vi "CV_CB_main.vi"() -> ()   [LabVIEW 2021]
uses:
  C:/Users/User/Documents/Published_files/thorlabs_files/Thorlabs.MotionControl.Controls.dll
  thorlabs_files/Thorlabs.MotionControl.Controls.dll
  C:/Users/User/Documents/Published_files/thorlabs_files/ThorLabs.MotionControl.Benchtop.DCServoCLI.dll
  thorlabs_files/ThorLabs.MotionControl.Benchtop.DCServoCLI.dll
  C:/Users/User/Documents/Published_files/thorlabs_files/ThorLabs.MotionControl.KCube.DCServoCLI.dll
  thorlabs_files/ThorLabs.MotionControl.KCube.DCServoCLI.dll
  C:/Users/User/Documents/Published_files/thorlabs_files/Thorlabs.MotionControl.IntegratedStepperMotorsCLI.dll
  thorlabs_files/Thorlabs.MotionControl.IntegratedStepperMotorsCLI.dll
  <vilib>/Utility/file.llb/Read Delimited Spreadsheet (DBL).vi
  <vilib>/Utility/file.llb/Write Delimited Spreadsheet (DBL).vi
  <vilib>/ptbypt/NI_PtbyPt.lvlib
panel:
  in  "Use the last scan":bool
  out "Lumedica report 2":string
  in  "saveing method 2":string(combo)="SaveQueueImages"
  out "large_C":bool
  out "last Z":dbl format="%#.6g"
  in  "Pause Button":bool
  in  "Abort craniotomy":bool
  out "Going to perfrom a craniotomy":bool
  in  "Z-bias in pixels":dbl
  in  "feedrate (mm/s)":dbl=1.0
  out "TERMINATE":bool
  out "thickness":dbl
  out "calibration_pos":dbl[][](array[numeric])
  in  "Drilling type":i64(ring) items=["Constant remaining thickness", "Burr holes", "Constant trench depth"]
  in  "Refractive index":dbl=1.6
  in  "Previous Button":bool
  in  "Go to OCT site":bool
  in  "shut down":bool
  out "End":bool=TRUE
  out "Correction matrix":dbl[](array[numeric])
  out "Lumedica report":string
  in  "saveing method":string(combo)="SaveQueueImages"
  out "OCT_imaging_position":dbl[](array[numeric])
  in  "start OCT":bool
  out "OCT_on":bool
  out "X-stage Control":refnum<k24>
  out "X stage properties":refnum<k24>
  in  "LongTravelStageControl":refnum<k24>(container)
  out "Drill-Z-stage Control":refnum<k24>
  out "OCT-Z-stage-control":refnum<k24>
  out "Y-stage Control":refnum<k24>
  out "Y-stage properties":refnum<k24>
  out "Driller-Z-stage-Properties":refnum<k24>
  out "OCT-Z stage-properites":refnum<k24>
  in  "Trajectory":dbl[][](array[numeric])
  out "Velocity":T1(graph)
  out "position":T1(graph)
  in  "Driller Z- stage":refnum<k24>(container)
  in  "Y stage":refnum<k24>(container)
  in  "OCT Z-stage":refnum<k24>(container)
  # "Step Specified Controls"
  # "General Controls"
  # "Moving the stereotax to the OCT stage"
  # "OCT scanning"
  # "Moving to the surgery station"
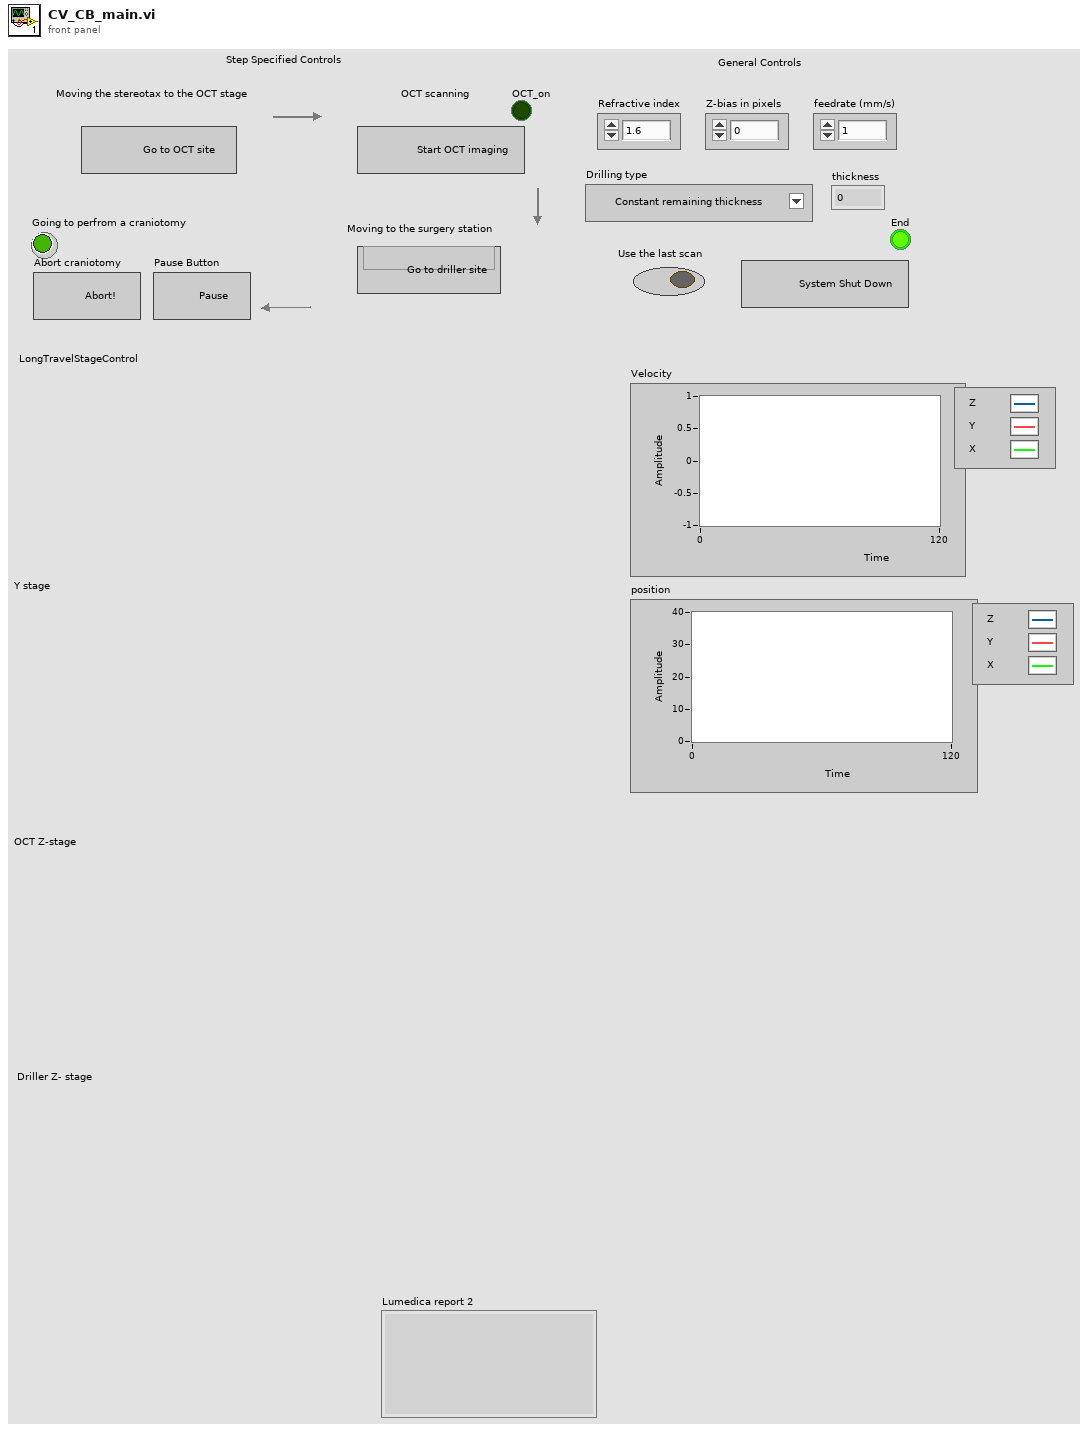
[diagram p1: front panel]
types:
  T1 = cluster{"[0]":dbl, "[1]":dbl, "[2]":dbl, "[3]":dbl, "[4]":dbl, "[5]":dbl, "[6]":dbl, "[7]":dbl, "[8]":dbl}
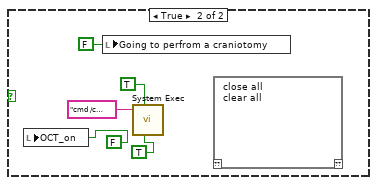
[diagram p2: hidden frame]
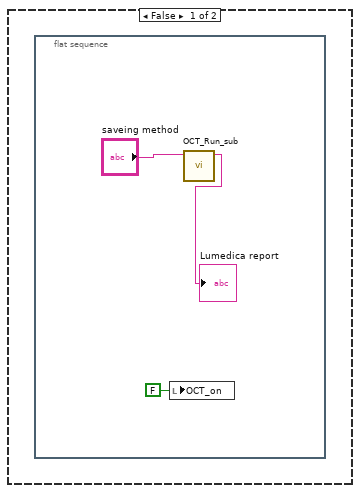
[diagram p5: hidden frame]
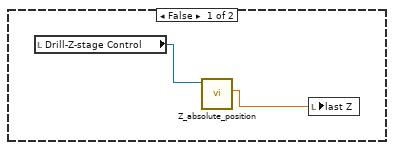
[diagram p9: hidden frame]
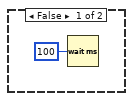
[diagram p10: hidden frame]
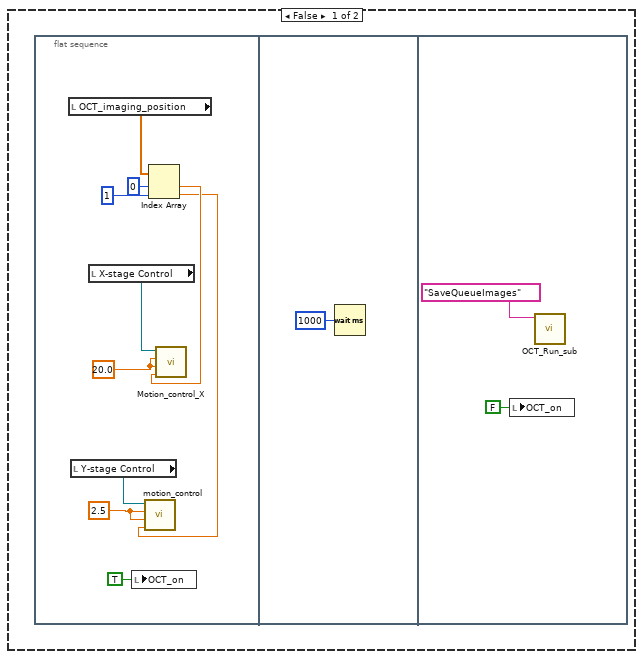
[diagram p12: hidden frame]
diagram:
  n1 = flat-sequence {
    frame #0 {
      # "Initiate all actuators"
      n2 = local write "End"(FALSE ("End")) -> ()
      n3 = property class="LongTravelStageControl"(reference="LongTravelStageControl", "SerialNumber"="45285094") -> (reference out=w25:refnum<k24>)  [unwired: 1 in, 1 out]
      n4 = property class="BenchtopDCServoControl"(reference="Y stage", "SerialNumber"="105278474") -> (reference out=w34:refnum<k24>)  [unwired: 1 in, 1 out]
      n5 = property class="KCubeDCServoControl"(reference="Driller Z- stage", "SerialNumber"="27260819") -> (reference out=w36:refnum<k24>)  [unwired: 1 in, 1 out]
      n6 = property class="KCubeDCServoControl"(reference="OCT Z-stage", "SerialNumber"="27261776") -> (reference out=w39:refnum<k24>)  [unwired: 1 in, 1 out]
      n7 = invoke class="LongTravelStageControl" method="CreateDevice"(reference=w25) -> (reference out=w24:refnum<k24>)  [unwired: 2 in, 2 out]
      n8 = invoke class="BenchtopDCServoControl" method="CreateDevice"(reference=w34) -> (reference out=w31:refnum<k24>)  [unwired: 2 in, 2 out]
      n9 = invoke class="KCubeDCServoControl" method="CreateDevice"(reference=w39) -> (reference out=w37:refnum<k24>)  [unwired: 2 in, 2 out]
      n10 = invoke class="KCubeDCServoControl" method="CreateDevice"(reference=w36) -> (reference out=w32:refnum<k24>)  [unwired: 2 in, 2 out]
      n11 = property class="LongTravelStageControl"(reference=w24) -> (reference out=w23:refnum<k24>, "Device"=w16:refnum<k24>)  [unwired: 1 in, 1 out]
      n12 = invoke class="IntegratedStepperMotor" method="SetBacklash"(reference=w16, "backlash"=0.002) -> ()  [unwired: 2 in, 4 out]
      n13 = property class="KCubeDCServoControl"(reference=w37) -> (reference out=w30:refnum<k24>, "Device"=w11:refnum<k24>)  [unwired: 1 in, 1 out]
      n14 = property class="BenchtopDCServoControl"(reference=w31) -> (reference out=w28:refnum<k24>, "BenchtopDCServo"=w14:refnum<k24>)  [unwired: 1 in, 1 out]
      n15 = invoke class="DCServoChannel" method="SetBacklash"(reference=w14, "backlash"=0.0) -> ()  [unwired: 2 in, 4 out]
      n16 = property class="KCubeDCServoControl"(reference=w32) -> (reference out=w29:refnum<k24>, "Device"=w27:refnum<k24>)  [unwired: 1 in, 1 out]
      n17 = invoke class="KCubeDCServo" method="SetBacklash"(reference=w27, "backlash"=0.007) -> ()  [unwired: 2 in, 4 out]
      n18 = invoke class="DCServoChannel" method="EnableDevice"(reference=w14) -> ()  [unwired: 2 in, 3 out]
      n19 = local write "OCT-Z stage-properites"(w30) -> ()
      n20 = local write "OCT-Z-stage-control"(w11) -> ()
      n21 = invoke class="KCubeDCServo" method="SetBacklash"(reference=w11, "backlash"=0.007) -> ()  [unwired: 2 in, 4 out]
      n22 = invoke class="IntegratedStepperMotor" method="EnableDevice"(reference=w16) -> ()  [unwired: 2 in, 3 out]
      n23 = local write "X stage properties"(w23) -> ()
      n24 = local write "X-stage Control"(w16) -> ()
      n25 = local write "Y-stage properties"(w28) -> ()
      n26 = local write "Y-stage Control"(w14) -> ()
      n27 = local write "Driller-Z-stage-Properties"(w29) -> ()
      n28 = local write "Drill-Z-stage Control"(w27) -> ()
    }
    frame #1 {
      # "Ready to take mouse to the imaging post"
      n29 = local read "Drill-Z-stage Control"() -> (w44:refnum<k24>)
      n30 = local write "OCT_on"(FALSE ("OCT_on")) -> ()
      n31 = call "motion control_Z.vi"("position"=0.0, "acceleration"=2.0, "maxVelocity"=2.0, ".NET Refnum in"=w44) -> ()  [unwired: 1 in, 1 out]
      n32 = call <vilib>:"System Exec.vi"("run minimized? (F)"=TRUE, "wait until completion? (T)"=TRUE, "command line"="cmd /c taskkill /IM OctEngine.exe") -> ()  [unwired: 5 in, 4 out]
      n33 = Two Button Dialog(message="Ready to move the mouse to OCT stage?", 1:"Nope! wait" ("F button name (\"Cancel\")"), 2:"Yes!" ("T button name (\"OK\")")) -> (T button?=w48:bool)
      n34 = while {
        tunnel: w48 -> [w52]
        stop <- w54 stop-if-true
        n35 = Or(x="Go to OCT site", y=w52) -> (x .or. y?=w54:bool)
      }
    }
    frame #2 {
      w68 = 3.0 ("maxVelocity")
      w73 = 20.0 ("maxVelocity")
      # "Move X actuator to 285mm"
      n36 = local read "X-stage Control"() -> (w74:refnum<k24>)
      n37 = call <vilib>:"Application Directory.vi"() -> ("Application Directory"=w62:path)
      n38 = local read "Y-stage Control"() -> (w70:refnum<k24>)
      n39 = local read "OCT-Z-stage-control"() -> (w69:refnum<k24>)
      n40 = Build Path(base path=w62, name or relative path=path "temp_files/Calibration_imaging_position.txt" ("file path (dialog if empty)")) -> (appended path=w63:path)
      n41 = call-poly <vilib>:"Read Delimited Spreadsheet.vi"("file path (dialog if empty)"=w63) -> ("all rows"=w60:dbl[][])  [unwired: 9 in, 5 out]
      n42 = local write "calibration_pos"(w60) -> ()
      n43 = Index Array(array=w60, index (row)=0, index (col)=1 ("disabled index (col)")) -> (element=w55:dbl)
      n44 = Index Array(array=w60, index (row)=0, index (col)=0 ("disabled index (col)")) -> (element=w61:dbl)
      n45 = call "Motion_control_X.vi"(".NET Refnum in"=w74, "maxVelocity"=w73, "acceleration"=w73, "position"=w61) -> ()  [unwired: 6 in, 1 out]
      n46 = Index Array(array=w60, index (row)=0 ("disabled index (row)"), index (col)=2 ("disabled index (col)")) -> (element=w66:dbl)
      n47 = call "motion_control.vi"("position"=w55, "acceleration"=5.0, "maxVelocity"=2.5, ".NET Refnum in"=w70) -> ()  [unwired: 1 in, 1 out]
      n48 = call "motion control_Z.vi"("position"=w66, "acceleration"=w68, "maxVelocity"=w68, ".NET Refnum in"=w69) -> ()  [unwired: 1 in, 1 out]
    }
    frame #3 {
      n49 = Two Button Dialog(message="What is the size of your FOV?", 1:"Less than 5 mm2" ("F button name (\"Cancel\")"), 2:"More than 5 mm2" ("T button name (\"OK\")")) -> (T button?=w75:bool)
      n50 = local write "large_C"(w75) -> ()
    }
    frame #4 {
      # "Manually adjust the imaging setp"
      n51 = while {
        stop <- w82 stop-if-true
        n52 = One Button Dialog(message="Adjust the sample position under the scanner and hit \"Take OCT image\" in labview", button name ("OK")="OK") -> (true=w82:bool)
      }
      n53 = Wait (ms)(milliseconds to wait=u32 1000) -> ()  [unwired: 1 out]
    }
    frame #5 {
      # "Show the USB camera and the FOV"
      n54 = local read "large_C"() -> (w84:bool)
      n55 = call <vilib>:"Application Directory.vi"() -> ("Application Directory"=w85:path)
      n56 = Boolean To (0,1)(Boolean=w84) -> (0, 1=w83:i16)
      n57 = script code="load([path,'\\temp_files\\pilot.mat'])\nif large>0\n     Xoff=110; Yoff=80;\nelse\n     Xoff=0; Yoff=0;\nend\nvid = videoinput('winvideo',OCT_cam);\nvidRes = vid.VideoResolution;\nnBands = vid.NumberOfBands; \n\nhFig=figure('Renderer', 'painters', 'Position', [1100 200 vidRes(1)/2+2*Xoff vidRes(2)]);\nhAxes = axes(hFig);\nhImage = image(hAxes, zeros(vidRes(2), vidRes(1)/2+2*Xoff, nBands)); \n\nsetappdata(hImage,'UpdatePreviewWindowFcn',@mypreview_fnc);\n\npreview(vid, hImage); \n% adding the OCT image boarders to the video\nhold on\ntext(-40,-35,'Make sure your ROI is in the green rectangle. if it is, just close the window','FontWeight','bold','FontSize',12)\n\nline([pilot(4,1)-Xoff pilot(1,1)+Xoff], [pilot(4,2)-Yoff pilot(1,2)-Yoff],'Color','g','LineWidth',3);\nline([pilot(3,1)-Xoff pilot(4,1)-Xoff], [pilot(3,2)+Yoff pilot(4,2)-Yoff],'Color','g','LineWidth',3);\nline([pilot(2,1)+Xoff pilot(3,1)-Xoff], [pilot(2,2)+Yoff pilot(3,2)+Yoff],'Color','g','LineWidth',3);\nline([pilot(1,1)+Xoff pilot(2,1)+Xoff], [pilot(1,2)-Yoff pilot(2,2)+Yoff],'Color','g','LineWidth',3);\n\n\nclear camObject;"("path"=w85, "large"=w83) -> ()  [unwired: 1 in, 1 out]
    }
    frame #6 {
      # "Acquire the stage positions during imaging"
      n58 = case shown="False" "Use the last scan" {
        frame False {
          n59 = while {
            tunnel: [w100] -> w88
            tunnel: [w99] -> w87
            tunnel: [w98] -> w94
            stop <- w96 stop-if-true
            n60 = local read "OCT-Z-stage-control"() -> (w101:refnum<k24>)
            n61 = local read "Y-stage Control"() -> (w102:refnum<k24>)
            n62 = local read "X-stage Control"() -> (w103:refnum<k24>)
            n63 = local read "TERMINATE"() -> (w95:bool)
            n64 = call "Y_absolute_position.vi"(".NET Refnum in"=w102) -> ("Numeric"=w99:dbl)  [unwired: 9 in, 1 out]
            n65 = Or(x=w95, y="start OCT") -> (x .or. y?=w96:bool)
            n66 = call "X-absolute_position.vi"(".NET Refnum in"=w103) -> ("Numeric"=w100:dbl)  [unwired: 9 in, 1 out]
            n67 = call "Z_absolute_position.vi"(".NET Refnum in"=w101) -> ("Numeric"=w98:dbl)  [unwired: 9 in, 1 out]
          }
          n68 = local write "OCT_on"(TRUE ("OCT_on")) -> ()
          n69 = Build Array(w88, w87, w94) -> (w93:dbl[])
          n70 = local write "OCT_imaging_position"(w93) -> ()
          n71 = call <vilib>:"Application Directory.vi"() -> ("Application Directory"=w91:path)
          n72 = Build Path(base path=w91, name or relative path=path "temp_files/imaging_position.txt" ("file path (dialog if empty)")) -> (appended path=w89:path)
          n73 = call-poly <vilib>:"Write Delimited Spreadsheet.vi"("file path (dialog if empty)"=w89, "1D data"=w93) -> ()  [unwired: 12 in, 2 out]
        }
        frame True {
        }
      }
    }
    frame #7 {
      n74 = local read "Use the last scan"() -> (w104:bool)
      n75 = case shown="False" w104 {
        frame False {
          # "Take the OCT image"
          n76 = local read "large_C"() -> (w105:bool)
          n77 = case shown="True" w105 {
            frame False {
              n78 = flat-sequence {
                frame #0 {
                  n79 = local write "OCT_on"(FALSE ("OCT_on")) -> ()
                  n80 = call "OCT_Run_sub.vi"("saveing method"="saveing method") -> ("Lumedica report"=→"Lumedica report":string)  [unwired: 10 in]
                }
              }
            }
            frame True {
              w110 = -2.25 ("element")
              w111 = 2.25 ("element")
              w113 = -2.0 ("element")
              w114 = 2.0 ("element")
              # "Shifts need in Y direction for each\nquarter of the big scan with respect to the center"
              # "Shifts need in X direction for each\nquarter of the big scan with respect to the center"
              # "make sure it is 4"
              n81 = Build Array(w111, w110, w110, w111) -> (w109:dbl[])
              n82 = Build Array(w114, w114, w113, w113) -> (w112:dbl[])
              n83 = for {
                N: 4 -> [_]
                tunnel: w112 -> [w118] mode=indexing
                tunnel: w109 -> [w117] mode=indexing
                n84 = flat-sequence {
                  tunnel: w118 -> [w123]
                  tunnel: w117 -> [w120]
                  frame #0 {
                    w128 = 2.0 ("maxVelocity")
                    w129 = 2.0 ("maxVelocity")
                    # "move to the target quarter"
                    n85 = local read "OCT_imaging_position"() -> (w127:dbl[])
                    n86 = local read "X-stage Control"() -> (w131:refnum<k24>)
                    n87 = local read "Y-stage Control"() -> (w130:refnum<k24>)
                    n88 = Index Array(array=w127, index #1=0 ("index"), index #2=1 ("index")) -> (element #1=w124:dbl, element #2=w121:dbl)
                    n89 = Add(x=w124, y=w123) -> (x+y=w122:dbl)
                    n90 = Add(x=w121, y=w120) -> (x+y=w119:dbl)
                    n91 = call "motion_control.vi"("position"=w119, "acceleration"=w128, "maxVelocity"=w128, ".NET Refnum in"=w130) -> ()  [unwired: 1 in, 1 out]
                    n92 = call "Motion_control_X.vi"(".NET Refnum in"=w131, "maxVelocity"=w129, "acceleration"=w129, "position"=w122) -> ()  [unwired: 6 in, 1 out]
                  }
                  frame #1 {
                    n93 = Wait (ms)(milliseconds to wait=u32 1000) -> ()  [unwired: 1 out]
                  }
                  frame #2 {
                    # "Take OCT stack of the quarter"
                    n94 = call "OCT_Run_sub.vi"("saveing method"="saveing method 2") -> ("Lumedica report"=→"Lumedica report 2":string)  [unwired: 10 in]
                  }
                }
              }
              n95 = local write "OCT_on"(FALSE ("OCT_on")) -> ()
            }
          }
        }
        frame True {
        }
      }
    }
    frame #8 {
      # "Try to close the opened video windoe"
      # "Close lumedica and open video windows"
      n96 = script code="close all"() -> ()  [unwired: 1 in, 1 out]
      n97 = call <vilib>:"System Exec.vi"("run minimized? (F)"=TRUE, "wait until completion? (T)"=TRUE, "command line"="cmd /c taskkill /IM OctEngine.exe") -> ()  [unwired: 5 in, 4 out]
    }
    frame #9 {
      # "This address should be tha same as where OCT saves scans"
      # "Calculating the first path"
      n98 = local read "Z-bias in pixels"() -> (w141:dbl)
      n99 = local read "large_C"() -> (w139:bool)
      n100 = call "File Dialog2"() -> ("selected path"=w140:path)  [unwired: 12 in, 3 out]
      n101 = local write "Going to perfrom a craniotomy"(TRUE ("Going to perfrom a craniotomy")) -> ()
      n102 = local read "Drilling type"() -> (w145:i64)
      n103 = local read "calibration_pos"() -> (w142:dbl[][])
      n104 = call "Calculate_drilling_path.vi"("calibration_pos"=w142, "Refractive index of the sample"="Refractive index", "Drilling type"=w145, "Large_C"=w139, "Z-bias in pixels"=w141, "Drilling path"=w140, "file path (dialog if empty)"=path "C:/Users/Public/Documents/Lumedica/OctEngine/Data") -> ("depth"=→"thickness":dbl)  [unwired: 4 in]
    }
    frame #10 {
      n105 = disable-structure shown="Disabled" {
        frame Disabled {
          n106 = Path To String(path=path "C:/Users/Public/Documents/Lumedica/OctEngine/Data" ("file path (dialog if empty)")) -> (string=w155:string)
          n107 = Concatenate Strings("cmd /k explorer.exe  " ("string"), w155, "\\figures" ("string")) -> (w153:string)
          n108 = call <vilib>:"System Exec.vi"("run minimized? (F)"=TRUE, "wait until completion? (T)"=FALSE, "command line"=w153) -> ()  [unwired: 5 in, 4 out]
        }
        frame Enabled {
        }
      }
      n109 = Two Button Dialog(message="Ready to move the mouse to drilling  stage?", 1:"Nope! wait" ("F button name (\"Cancel\")"), 2:"Yes!" ("T button name (\"OK\")")) -> (T button?=w147:bool)
      n110 = while {
        tunnel: w147 -> [w159]
        stop <- w160 stop-if-true
        n111 = Or(x=w159, y="Previous Button") -> (x .or. y?=w160:bool)
      }
    }
    frame #11 {
      w166 = 20.0 ("maxVelocity")
      # "Move the stage to the drilling site"
      n112 = local read "Y-stage Control"() -> (w162:refnum<k24>)
      n113 = local read "X-stage Control"() -> (w161:refnum<k24>)
      n114 = call "Motion_control_X.vi"(".NET Refnum in"=w161, "maxVelocity"=w166, "acceleration"=w166, "position"=17.0) -> ()  [unwired: 6 in, 1 out]
      n115 = call "motion_control.vi"("position"=10.0, "acceleration"=5.0, "maxVelocity"=2.5, ".NET Refnum in"=w162) -> ()  [unwired: 1 in, 1 out]
    }
    frame #12 {
      # "turn on the drill camera"
      n116 = call <vilib>:"Application Directory.vi"() -> ("Application Directory"=w168:path)
      n117 = script code="load([path,'\\temp_files\\pilot.mat'])\ncrop_pixels=100;\nvid = videoinput('winvideo',Drill_cam);\nvidInfo = imaqhwinfo(vid);\nvidRes = vid.VideoResolution;\nnBands = vid.NumberOfBands; \nhFig=figure('Renderer', 'painters', 'Position', [1200 200 vidRes(1)/2 vidRes(2)/2]);\nhAxes = axes(hFig);\nhImage = image(hAxes, zeros(vidRes(2), vidRes(1), nBands)); \n%setappdata(hImage,'UpdatePreviewWindowFcn',@mypreview_fnc);\npreview(vid, hImage); \n% adding the OCT image boarders to the video\nhold on\ntext(-40,-35,'Drilling FOV','FontWeight','bold','FontSize',12)\n\nclear camObject;"("path"=w168) -> ()  [unwired: 1 in, 1 out]
    }
    frame #13 {
      # "Ready for drilling!"
      n118 = while {
        stop <- w171 stop-if-true
        n119 = One Button Dialog(message="Drop sailine on top of  the skull , TURN ON THE DRILLERTand press ok when you are ready", button name ("OK")="OK") -> (true=w171:bool)
      }
    }
    frame #14 {
      n120 = while {
        stop <- w180 stop-if-true
        n121 = flat-sequence {
          tunnel: [w181] -> w179
          tunnel: w179 -> [w185]
          tunnel: [w186] -> w178
          tunnel: [w185] -> w176
          tunnel: w178 -> [w204]
          tunnel: [w203] -> w177
          tunnel: w176 -> [w203]
          tunnel: w177 -> [w209]
          tunnel: [w208] -> w175
          tunnel: [w207] -> w174
          tunnel: w175 -> [w224]
          tunnel: w174 -> [w223]
          tunnel: [w258] -> w173
          tunnel: w173 -> [w262]
          tunnel: [w262] -> w172
          frame #0 {
            # "read the calculated drilling path"
            n122 = call <vilib>:"Application Directory.vi"() -> ("Application Directory"=w184:path)
            n123 = Build Path(base path=w184, name or relative path=path "temp_files/C_TD_path.txt" ("file path (dialog if empty)")) -> (appended path=w183:path)
            n124 = call-poly <vilib>:"Read Delimited Spreadsheet.vi"("file path (dialog if empty)"=w183) -> ("all rows"=w181:dbl[][])  [unwired: 9 in, 5 out]
          }
          frame #1 {
            w197 = 2.0 ("maxVelocity")
            w201 = 20.0 ("maxVelocity")
            # "Move to the first poin-0.5 mm up"
            n125 = local read "Drill-Z-stage Control"() -> (w199:refnum<k24>)
            n126 = Index Array(array=w185, index (row)=0) -> (element=w193:dbl[])  [unwired: 1 in]
            n127 = local read "X-stage Control"() -> (w202:refnum<k24>)
            n128 = Index Array(array=w193, index #1=0 ("index"), index #2=1 ("index"), index #3=2 ("index")) -> (element #1=w187:dbl, element #2=w188:dbl, element #3=w186:dbl)
            n129 = Subtract(x=w186, y=0.5) -> (x-y=w200:dbl)
            n130 = local read "Y-stage Control"() -> (w196:refnum<k24>)
            n131 = call "motion control_Z.vi"("position"=w200, "acceleration"=w197, "maxVelocity"=w197, ".NET Refnum in"=w199) -> ()  [unwired: 1 in, 1 out]
            n132 = call "motion_control.vi"("position"=w188, "acceleration"=5.0, "maxVelocity"=2.5, ".NET Refnum in"=w196) -> ()  [unwired: 1 in, 1 out]
            n133 = call "Motion_control_X.vi"(".NET Refnum in"=w202, "maxVelocity"=w201, "acceleration"=w201, "position"=w187) -> ()  [unwired: 6 in, 1 out]
          }
          frame #2 {
            w205 = 0.25 ("maxVelocity")
            # "Drill down the first point"
            n134 = local read "Drill-Z-stage Control"() -> (w206:refnum<k24>)
            n135 = call "motion control_Z.vi"("position"=w204, "acceleration"=w205, "maxVelocity"=w205, ".NET Refnum in"=w206) -> ()  [unwired: 1 in, 1 out]
          }
          frame #3 {
            # "calculate speeds and positions"
            n136 = disable-structure shown="Disabled" {
              disable-tunnel: w209 -> [w211 _]
              frame Disabled {
                n137 = script code="ratio=1;\ndata=C_TD_path(:,1:3)';\n[q, qd, qdd, tvec, pp] = trapveltraj(data,length(C_TD_path));\ncoef=pp{1,1}.coefs;\naccX=2*coef(4:9:end,1);\naccY=2*coef(5:9:end,1);\naccZ=2*coef(6:9:end,1);\nmVelX=coef(7:9:end,2);\nmVelY=coef(8:9:end,2);\nmVelZ=coef(9:9:end,2);\nmVel=ratio*abs([mVelX mVelY mVelZ]);\nmVel(mVel<0.02)=0.02;\nacc=(ratio^2)*abs([accX accY accZ]);\nacc(acc<0.02)=0.02;\nTime=pp{1,1}.breaks;\nTime=Time(2:3:end);\nWTime=Time(2:end)-Time(1:end-1);\nsteps=length(WTime);\ndata=data(:,2:end)';"("C_TD_path"=w211) -> ("mVel"=w212:dbl[][], "acc"=w213:dbl[][], "data"=w210:dbl[][])  [unwired: 1 in, 2 out]
                n138 = call <vilib>:"Application Directory.vi"() -> ("Application Directory"=w222:path)
                n139 = call <vilib>:"Application Directory.vi"() -> ("Application Directory"=w221:path)
                n140 = call <vilib>:"Application Directory.vi"() -> ("Application Directory"=w220:path)
                n141 = Build Path(base path=w222, name or relative path=path "temp_files/F_a_log.txt" ("file path (dialog if empty)")) -> (appended path=w214:path)
                n142 = Build Path(base path=w221, name or relative path=path "temp_files/F_p_log.txt" ("file path (dialog if empty)")) -> (appended path=w216:path)
                n143 = Build Path(base path=w220, name or relative path=path "temp_files/F_v_log.txt" ("file path (dialog if empty)")) -> (appended path=w219:path)
                n144 = call-poly <vilib>:"Write Delimited Spreadsheet.vi"("file path (dialog if empty)"=w219, "2D data"=w212) -> ()  [unwired: 12 in, 2 out]
                n145 = call-poly <vilib>:"Write Delimited Spreadsheet.vi"("file path (dialog if empty)"=w214, "2D data"=w213) -> ()  [unwired: 12 in, 2 out]
                n146 = call-poly <vilib>:"Write Delimited Spreadsheet.vi"("file path (dialog if empty)"=w216, "2D data"=w210) -> ()  [unwired: 12 in, 2 out]
              }
              frame Enabled {
              }
            }
            n147 = script code="data=C_TD_path(:,1:3)';\ndata=data(:,2:end)';\nsteps=length(data);"("C_TD_path"=w209) -> ("steps"=w208:dbl, "data"=w207:dbl[][])  [unwired: 1 in, 1 out]
          }
          frame #4 {
            # "actuators moving"
            n148 = for {
              N: w224 -> [_]
              tunnel: w223 -> [w234] mode=indexing
              stop <- "Abort craniotomy" stop-if-true
              n149 = case shown="True" "Pause Button" {
                frame False {
                  n150 = local read "Drill-Z-stage Control"() -> (w239:refnum<k24>)
                  n151 = call "Z_absolute_position.vi"(".NET Refnum in"=w239) -> ("Numeric"=w238:dbl)  [unwired: 9 in, 1 out]
                  n152 = local write "last Z"(w238) -> ()
                }
                frame True {
                  w240 = 2.0 ("maxVelocity")
                  # "bring driller up for the moment"
                  n153 = flat-sequence {
                    frame #0 {
                      n154 = while {
                        stop <- w247 stop-if-true
                        n155 = One Button Dialog(message="Are you ready to go back?", button name ("OK")="Yup!") -> (true=w247:bool)
                      }
                    }
                    frame #1 {
                      w251 = 1.1 ("maxVelocity")
                      n156 = local read "Drill-Z-stage Control"() -> (w249:refnum<k24>)
                      n157 = local read "last Z"() -> (w250:dbl)
                      n158 = call "motion control_Z.vi"("position"=w250, "acceleration"=w251, "maxVelocity"=w251, ".NET Refnum in"=w249) -> ()  [unwired: 1 in, 1 out]
                    }
                  }
                  n159 = local read "Drill-Z-stage Control"() -> (w245:refnum<k24>)
                  n160 = call "Z_absolute_position.vi"(".NET Refnum in"=w245) -> ("Numeric"=w243:dbl, ".NET Refnum out"=w244:refnum<k24>)  [unwired: 9 in]
                  n161 = Subtract(x=w243, y=10.0) -> (x-y=w241:dbl)
                  n162 = call "motion control_Z.vi"("position"=w241, "acceleration"=w240, "maxVelocity"=w240, ".NET Refnum in"=w244) -> ()  [unwired: 1 in, 1 out]
                }
              }
              n163 = local read "Drill-Z-stage Control"() -> (w230:refnum<k24>)
              n164 = local read "feedrate (mm/s)"() -> (w227:dbl)
              n165 = local read "X-stage Control"() -> (w229:refnum<k24>)
              n166 = local read "Y-stage Control"() -> (w228:refnum<k24>)
              n167 = Index Array(array=w234, index #1=0 ("index"), index #2=1 ("index"), index #3=2 ("index")) -> (element #1=w233:dbl, element #2=w232:dbl, element #3=w231:dbl)
              n168 = call "motion_control.vi"("position"=w232, "acceleration"=w227, "maxVelocity"=w227, ".NET Refnum in"=w228) -> ()  [unwired: 1 in, 1 out]
              n169 = call "Motion_control_X.vi"(".NET Refnum in"=w229, "maxVelocity"=w227, "acceleration"=w227, "position"=w233) -> ()  [unwired: 6 in, 1 out]
              n170 = call "motion control_Z.vi"("position"=w231, "acceleration"=w227, "maxVelocity"=w227, ".NET Refnum in"=w230) -> ()  [unwired: 1 in, 1 out]
            }
          }
          frame #5 {
            w254 = 2.0 ("acceleration")
            # "Move up the drillbit after finishing"
            n171 = local read "Drill-Z-stage Control"() -> (w257:refnum<k24>)
            n172 = call "Z_absolute_position.vi"(".NET Refnum in"=w257) -> ("Numeric"=w253:dbl, ".NET Refnum out"=w256:refnum<k24>)  [unwired: 9 in]
            n173 = Subtract(x=w253, y=10.0) -> (x-y=w255:dbl)
            n174 = call "motion control_Z.vi"("position"=w255, "acceleration"=w254, "maxVelocity"=w254, ".NET Refnum in"=w256) -> ()  [unwired: 1 in, 1 out]
          }
          frame #6 {
            # "Asking if extra craniotomies are needed"
            n175 = Two Button Dialog(message="would you like to perform another craniotomy?", 1:"Nope. Done!" ("F button name (\"Cancel\")"), 2:"Yes!" ("T button name (\"OK\")")) -> (T button?=w258:bool)
            n176 = local write "Going to perfrom a craniotomy"(w258) -> ()
          }
          frame #7 {
            n177 = case shown="True" w262 {
              frame False {
                n178 = Wait (ms)(milliseconds to wait=u32 100) -> ()  [unwired: 1 out]
              }
              frame True {
                n179 = flat-sequence {
                  tunnel: [w266] -> w264
                  tunnel: w264 -> [w268]
                  frame #0 {
                    n180 = call "File Dialog"("prompt"="Choose the drilling path") -> ("selected path"=w266:path)  [unwired: 11 in, 3 out]
                  }
                  frame #1 {
                    n181 = local read "Z-bias in pixels"() -> (w272:dbl)
                    n182 = local read "large_C"() -> (w267:bool)
                    n183 = local read "Drilling type"() -> (w270:i64)
                    n184 = local read "Refractive index"() -> (w273:dbl)
                    n185 = local read "calibration_pos"() -> (w274:dbl[][])
                    n186 = call "Calculate_drilling_path.vi"("calibration_pos"=w274, "Refractive index of the sample"=w273, "Drilling type"=w270, "Large_C"=w267, "Z-bias in pixels"=w272, "Drilling path"=w268, "file path (dialog if empty)"=path "C:/Users/Public/Documents/Lumedica/OctEngine/Data") -> ("depth"=w271:dbl)  [unwired: 4 in]
                    n187 = local write "thickness"(w271) -> ()
                  }
                }
              }
            }
          }
        }
        n188 = Not(x=w172) -> (.not. x?=w180:bool)
      }
    }
    frame #15 {
      w275 = 2.0 ("position")
      n189 = local read "Drill-Z-stage Control"() -> (w277:refnum<k24>)
      n190 = call "motion control_Z.vi"("position"=0.0 ("maxVelocity"), "acceleration"=w275, "maxVelocity"=w275, ".NET Refnum in"=w277) -> ()  [unwired: 1 in, 1 out]
    }
    frame #16 {
      n191 = Two Button Dialog(message="Would you like to check the drilled path", 1:"No" ("F button name (\"Cancel\")"), 2:"Yes!" ("T button name (\"OK\")")) -> (T button?=w278:bool)
      n192 = case shown="True" w278 {
        frame False {
        }
        frame True {
          n193 = local read "large_C"() -> (w282:bool)
          n194 = case shown="True" w282 {
            frame False {
              n195 = flat-sequence {
                frame #0 {
                  w291 = 2.5 ("maxVelocity")
                  w292 = 20.0 ("maxVelocity")
                  n196 = local read "OCT_imaging_position"() -> (w288:dbl[])
                  n197 = local read "Y-stage Control"() -> (w289:refnum<k24>)
                  n198 = local read "X-stage Control"() -> (w290:refnum<k24>)
                  n199 = local write "OCT_on"(TRUE ("OCT_on")) -> ()
                  n200 = Index Array(array=w288, index #1=0 ("index"), index #2=1 ("index")) -> (element #1=w285:dbl, element #2=w284:dbl)
                  n201 = call "motion_control.vi"("position"=w284, "acceleration"=w291, "maxVelocity"=w291, ".NET Refnum in"=w289) -> ()  [unwired: 1 in, 1 out]
                  n202 = call "Motion_control_X.vi"(".NET Refnum in"=w290, "maxVelocity"=w292, "acceleration"=w292, "position"=w285) -> ()  [unwired: 6 in, 1 out]
                }
                frame #1 {
                  n203 = Wait (ms)(milliseconds to wait=u32 1000) -> ()  [unwired: 1 out]
                }
                frame #2 {
                  n204 = local write "OCT_on"(FALSE ("OCT_on")) -> ()
                  n205 = call "OCT_Run_sub.vi"("saveing method"="SaveQueueImages") -> ()  [unwired: 10 in, 1 out]
                }
              }
            }
            frame True {
              w299 = -2.25 ("element")
              w300 = 2.25 ("element")
              w301 = -2.0 ("element")
              w302 = 2.0 ("element")
              n206 = Build Array(w300, w299, w299, w300) -> (w297:dbl[])
              n207 = Build Array(w302, w302, w301, w301) -> (w298:dbl[])
              n208 = for {
                N: 4 -> [_]
                tunnel: w298 -> [w305] mode=indexing
                tunnel: w297 -> [w304] mode=indexing
                n209 = flat-sequence {
                  tunnel: w305 -> [w310]
                  tunnel: w304 -> [w308]
                  frame #0 {
                    w317 = 20.0 ("acceleration")
                    w318 = 2.5 ("acceleration")
                    n210 = local read "OCT_imaging_position"() -> (w314:dbl[])
                    n211 = local read "Y-stage Control"() -> (w316:refnum<k24>)
                    n212 = local read "X-stage Control"() -> (w315:refnum<k24>)
                    n213 = Index Array(array=w314, index #1=0 ("index"), index #2=1 ("index")) -> (element #1=w311:dbl, element #2=w307:dbl)
                    n214 = Add(x=w307, y=w308) -> (x+y=w306:dbl)
                    n215 = Add(x=w311, y=w310) -> (x+y=w309:dbl)
                    n216 = call "motion_control.vi"("position"=w306, "acceleration"=w318, "maxVelocity"=w318, ".NET Refnum in"=w316) -> ()  [unwired: 1 in, 1 out]
                    n217 = call "Motion_control_X.vi"(".NET Refnum in"=w315, "maxVelocity"=w317, "acceleration"=w317, "position"=w309) -> ()  [unwired: 6 in, 1 out]
                  }
                  frame #1 {
                    n218 = Wait (ms)(milliseconds to wait=u32 1000) -> ()  [unwired: 1 out]
                  }
                  frame #2 {
                    n219 = call "OCT_Run_sub.vi"() -> ()  [unwired: 11 in, 1 out]
                  }
                }
              }
              n220 = local write "OCT_on"(TRUE ("OCT_on")) -> ()
            }
          }
        }
      }
    }
    frame #17 {
      n221 = script code="clear camObject;\nclose all\nclearvars\npack;\nclear all"() -> ()  [unwired: 1 in, 1 out]
    }
    frame #18 {
      n222 = local write "OCT_on"(FALSE ("OCT_on")) -> ()
      n223 = local write "End"(TRUE) -> ()
    }
  }
  n224 = local read "OCT-Z stage-properites"() -> (w2:refnum<k24>)
  n225 = local read "OCT-Z stage-properites"() -> (w4:refnum<k24>)
  n226 = local read "X stage properties"() -> (w1:refnum<k24>)
  n227 = local read "Y-stage properties"() -> (w3:refnum<k24>)
  n228 = flat-sequence {
    tunnel: w4 -> [w328]
    tunnel: w3 -> [w327]
    tunnel: [w326] -> w10
    tunnel: [w330] -> w9
    tunnel: [w329] -> w8
    tunnel: w2 -> [w326]
    tunnel: [w325] -> w7
    tunnel: [w324] -> w6
    tunnel: w1 -> [w323]
    tunnel: [w322] -> w5
    tunnel: w10 -> [w368]
    tunnel: w9 -> [w369]
    tunnel: w8 -> [w370]
    tunnel: w7 -> [w367]
    tunnel: w6 -> [w366]
    tunnel: w5 -> [w365]
    frame #0 {
      n229 = while {
        tunnel: [w352] -> w330
        tunnel: w328 -> [w352]
        tunnel: w327 -> [w351]
        tunnel: [w351] -> w329
        tunnel: [w341] -> w325 mode=indexing
        tunnel: [w340] -> w324 mode=indexing
        tunnel: w323 -> [w339]
        tunnel: [w339] -> w322
        stop <- w331 stop-if-true
        w337 = u32 250 ("milliseconds to wait")
        w346 = 0.0 ("initial condition")
        n230 = local read "Drill-Z-stage Control"() -> (w342:refnum<k24>)
        n231 = local read "X-stage Control"() -> (w338:refnum<k24>)
        n232 = local read "Y-stage Control"() -> (w343:refnum<k24>)
        n233 = local read "End"() -> (w333:bool)
        n234 = call "Y_absolute_position.vi"(".NET Refnum in"=w343) -> ("Numeric"=w345:dbl)  [unwired: 9 in, 1 out]
        n235 = call "Z_absolute_position.vi"(".NET Refnum in"=w342) -> ("Numeric"=w344:dbl)  [unwired: 9 in, 1 out]
        n236 = call "X-absolute_position.vi"(".NET Refnum in"=w338) -> ("Numeric"=w335:dbl)  [unwired: 9 in, 1 out]
        n237 = Or(x="shut down", y=w333) -> (x .or. y?=w331:bool)
        "TERMINATE" <- w331
        n238 = case shown="False" w331 {
          frame False {
          }
          frame True {
            n239 = local write "OCT_on"(FALSE ("OCT_on")) -> ()
            n240 = local write "Going to perfrom a craniotomy"(FALSE ("Going to perfrom a craniotomy")) -> ()
            n241 = call <vilib>:"System Exec.vi"("run minimized? (F)"=TRUE, "wait until completion? (T)"=TRUE, "command line"="cmd /c taskkill /IM OctEngine.exe") -> ()  [unwired: 5 in, 4 out]
            n242 = script code="close all\nclear all"() -> ()  [unwired: 1 in, 1 out]
          }
        }
        n243 = call <vilib>:"Derivative x(t) PtByPt.vi"("dt"=w337, "initial condition"=w346, "x"=w344) -> ("dx/dt"=w348:dbl)  [unwired: 1 in, 1 out]
        n244 = call <vilib>:"Derivative x(t) PtByPt.vi"("dt"=w337, "initial condition"=w346, "x"=w344) -> ("dx/dt"=w347:dbl)  [unwired: 1 in, 1 out]
        n245 = call <vilib>:"Derivative x(t) PtByPt.vi"("dt"=w337, "initial condition"=0.0, "x"=w335) -> ("dx/dt"=w334:dbl)  [unwired: 1 in, 1 out]
        n246 = Build Array(w344, w345, w335) -> (w340:dbl[])
        n247 = Build Array(w347, w348, w334) -> (w341:dbl[])
        n248 = Array To Cluster(array=w340) -> (cluster=→"position":T1)
        n249 = Wait (ms)(milliseconds to wait=w337) -> ()  [unwired: 1 out]
        n250 = Array To Cluster(array=w341) -> (cluster=→"Velocity":T1)
      }
    }
    frame #1 {
      n251 = call <vilib>:"Application Directory.vi"() -> ("Application Directory"=w364:path)
      n252 = invoke class="BenchtopDCServoControl" method="CloseDevice"(reference=w370) -> ()  [unwired: 2 in, 3 out]
      n253 = invoke class="KCubeDCServoControl" method="CloseDevice"(reference=w369) -> ()  [unwired: 2 in, 3 out]
      n254 = invoke class="LongTravelStageControl" method="CloseDevice"(reference=w365) -> ()  [unwired: 2 in, 3 out]
      n255 = invoke class="KCubeDCServoControl" method="CloseDevice"(reference=w368) -> ()  [unwired: 2 in, 3 out]
      n256 = call <vilib>:"Application Directory.vi"() -> ("Application Directory"=w361:path)
      n257 = Build Path(base path=w361, name or relative path=path "temp_files/velocity log.txt" ("file path (dialog if empty)")) -> (appended path=w359:path)
      n258 = Build Path(base path=w364, name or relative path=path "temp_files/position log.txt" ("file path (dialog if empty)")) -> (appended path=w363:path)
      n259 = call-poly <vilib>:"Write Delimited Spreadsheet.vi"("file path (dialog if empty)"=w363, "2D data"=w366) -> ()  [unwired: 12 in, 2 out]
      n260 = Wait (ms)(milliseconds to wait=u32 100) -> ()  [unwired: 1 out]
      n261 = call-poly <vilib>:"Write Delimited Spreadsheet.vi"("file path (dialog if empty)"=w359, "2D data"=w367) -> ()  [unwired: 12 in, 2 out]
    }
    frame #2 {
      n262 = Stop(stop? (T)=TRUE) -> ()
    }
  }
  n263 = while {
    stop <- w372 stop-if-true
    n264 = local read "TERMINATE"() -> (w372:bool)
    n265 = Wait (ms)(milliseconds to wait=u32 20) -> ()  [unwired: 1 out]
  }
  n266 = while {
    stop <- FALSE stop-if-true
    n267 = local read "OCT_on"() -> (w375:bool)
    n268 = case shown="True" w375 {
      frame False {
      }
      frame True {
        n269 = Concatenate Strings("OctEngine.exe" ("string"), "\r\n") -> (w380:string)
        n270 = call <vilib>:"System Exec.vi"("run minimized? (F)"=FALSE, "wait until completion? (T)"=TRUE, "working directory"=path "C:/Program Files/Lumedica/OctEngine", "standard input"=w380, "command line"="cmd /k cd C:\\Program Files\\Lumedica\\OctEngine ") -> ()  [unwired: 3 in, 4 out]
      }
    }
  }
